vi "Fast Hilbert Transform.vi"(0 "X":dbl[](array[numeric])) -> (1 "Hilbert{X}":dbl[](array[numeric]), 2 "error":i32)   [LabVIEW 2024, in "NI_AALPro.lvlib"]
doc: "<p>Computes the fast Hilbert transform of the input sequence <strong>X</strong>.</p>"
uses:
  NI_AALPro.lvlib
  <resource>/lvanlys.dll
panel:
  # "Fast Hilbert Transform"
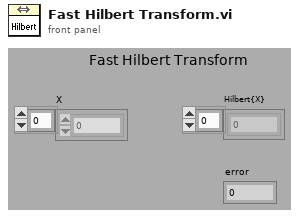
[diagram p1: front panel]
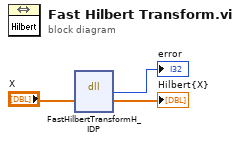
[diagram p0: block diagram]
diagram:
  n1 = dll-call lib="C:/Program Files (x86)/National Instruments/LabVIEW 2024/resource/lvanlys.*" fn="FastHilbertTransformH_IDP"("xH"="X") -> ("return type"=→"error":i32, "xH"=→"Hilbert{X}":dbl[])  [unwired: 5 in, 2 out]
